vi "Mouse Down.vi"(7 "Map Model in":refnum<class "Map Model.lvclass">, 8 "error in (no error)":errorcluster, 10 "Position":T1, 11 "Undoable Tool in":refnum<class "Undoable Tool.lvclass">) -> (0 "error out":errorcluster, 3 "Undoable Tool out":refnum<class "Undoable Tool.lvclass">, 5 "Map Model out":refnum<class "Map Model.lvclass">)   [LabVIEW 2020, in "Map Model.lvlib" / "Undoable Tool.lvclass"]
uses:
  Undoable Tool.lvclass
  <vilib>/Utility/miscctls.llb/LVPoint32TypeDef.ctl
  Map Model/Map Model.lvclass
  Undoable Tool.lvclass/Undoable Tool.ctl
  Tool/Tool.lvclass
panel:
  # "NOTICE -- YOU MUST LEAVE THIS NOTICE IN PLACE.\n\nCopyright (c) 2017, LIANG LIU Shawn.Liu.cn@gmail.com\nAll rights reserved.\n\nRedistribution and use in source and binary forms, with or without modification, are permitted provided that the following conditions are met:\n-Redistributions of source code must retain the above copyright notice, this list of conditions and the following disclaimer.\n-Redistributions in binary form must reproduce the above copyright notice, this list of conditions and the following disclaimer in the documentation and/or other materials provided with the distribution.\n-Neither the name of the eLp nor the names of its contributors may be used to endorse or promote products derived from this software without specific prior written permission.\n\nTHIS SOFTWARE IS PROVIDED BY THE COPYRIGHT HOLDERS AND CONTRIBUTORS \"AS IS\" AND ANY EXPRESS OR IMPLIED WARRANTIES, INCLUDING, BUT NOT LIMITED TO, THE IMPLIED WARRANTIES OF MERCHANTABILITY AND FITNESS FOR A PARTICULAR PURPOSE ARE DISCLAIMED. IN NO EVENT SHALL THE COPYRIGHT HOLDER OR CONTRIBUTORS BE LIABLE FOR ANY DIRECT, INDIRECT, INCIDENTAL, SPECIAL, EXEMPLARY, OR CONSEQUENTIAL DAMAGES (INCLUDING, BUT NOT LIMITED TO, PROCUREMENT OF SUBSTITUTE GOODS OR SERVICES; LOSS OF USE, DATA, OR PROFITS; OR BUSINESS INTERRUPTION) HOWEVER CAUSED AND ON ANY THEORY OF LIABILITY, WHETHER IN CONTRACT, STRICT LIABILITY, OR TORT (INCLUDING NEGLIGENCE OR OTHERWISE) ARISING IN ANY WAY OUT OF THE USE OF THIS SOFTWARE, EVEN IF ADVISED OF THE POSSIBILITY OF SUCH DAMAGE."
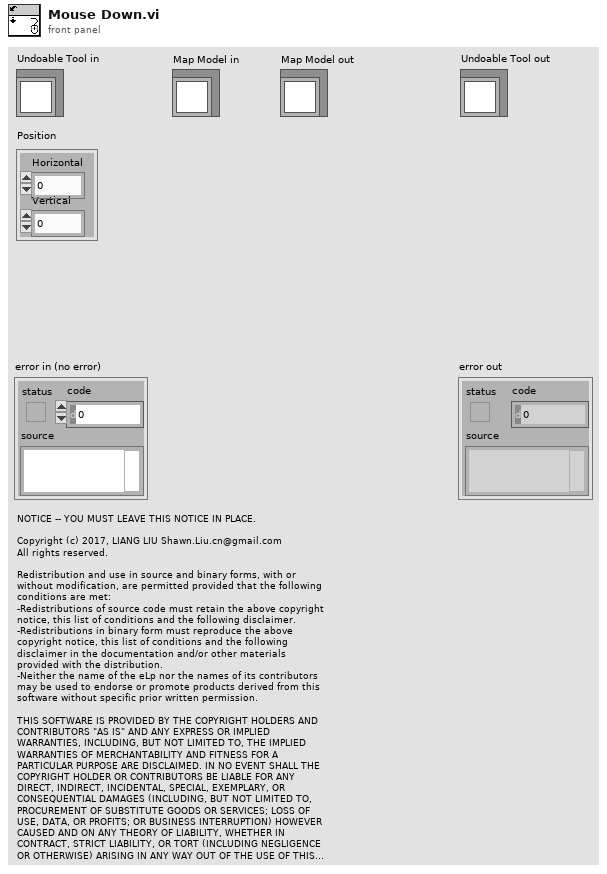
[diagram p1: front panel]
types:
  T1 = typedef "LVPoint32TypeDef.ctl" = cluster{"Horizontal":i32, "Vertical":i32}
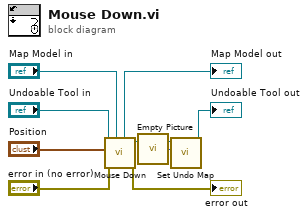
[diagram p0: block diagram]
diagram:
  n1 = call-parent "Mouse Down.vi"("Map Model in"="Map Model in", "error in (no error)"="error in (no error)", "Position"="Position", "Tool in"="Undoable Tool in") -> ("error out"=→"error out":errorcluster, "Tool out"=w5:refnum<class "Undoable Tool.lvclass">, "Map Model out"=→"Map Model out":refnum<class "Map Model.lvclass">)  [unwired: 5 in]
  n2 = call "Empty Picture"() -> ("empty picture"=w6:picture)
  n3 = call "Set Undo Map.vi"("Undo Map"=w6, "Undoable Tool in"=w5) -> ("Undoable Tool out"=→"Undoable Tool out":refnum<class "Undoable Tool.lvclass">)  [unwired: 9 in]
